vi "IsMultiDimensionArray.vi"(0 "Token Array":T1[](array[typedef]), 5 "Previous Index":i32) -> (4 "Is Nested Array?":bool)   [LabVIEW 2019, in "JsonToCluster.lvlib"]
doc: "It returns true, if the array has more then one dimension"
uses:
  JsonToCluster.lvlib
  _Controls/Tokens.ctl
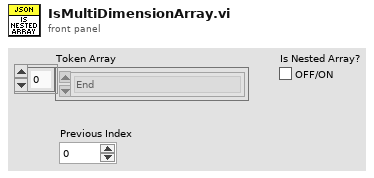
[diagram p1: front panel]
types:
  T1 = typedef "JsonToCluster.lvlib/Tokens.ctl" = enum16{"End", "Boolean", "Named Cluster", "Unnamed Cluster", "Array", "String", "Decimal", "FloatingPoint", "End Array", "End Cluster"}
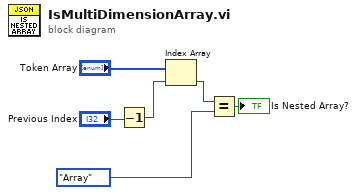
[diagram p0: block diagram]
diagram:
  n1 = Decrement(x="Previous Index") -> (x-1=w3:i32)
  n2 = Index Array(array="Token Array", index=w3) -> (element=w4:T1)
  n3 = Equal?(x=w4, y=Tokens."Array" ("x")) -> (x = y?=→"Is Nested Array?":bool)
